vi "2048_summon_ani.vi"(6 "speed":u32, 8 "Array in":refnum<vi>, 9 "c":u64, 10 "r":u64, 11 "element":i32) -> ()   [LabVIEW 2021]
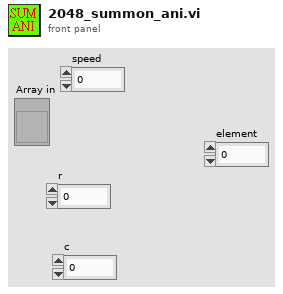
[diagram p1: front panel]
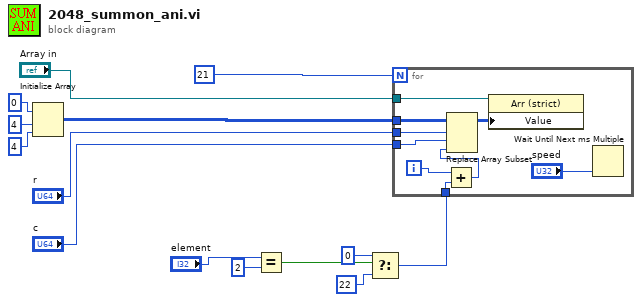
[diagram p0: block diagram]
diagram:
  n1 = Initialize Array(0 ("element"), 4 ("dimension size"), 4 ("dimension size")) -> (w14:i32[][])
  n2 = Equal?(x="element", y=2) -> (x = y?=w4:bool)
  n3 = Select(t=0, s=w4, f=22 ("t")) -> (s? t:f=w1:i32)
  n4 = for {
    N: 21 -> [_]
    tunnel: w14 -> [w23]
    tunnel: "c" -> [w21]
    tunnel: "r" -> [w20]
    tunnel: "Array in" -> [w19]
    tunnel: w1 -> [w17]
    i -> [w18]
    n5 = Add(x=w18, y=w17) -> (x+y=w16:i32)
    n6 = Replace Array Subset(array=w23, new element=w16, index (row)=w20, index (col)=w21) -> (w22:i32[][])
    n7 = property on="Property Node" class="Arr (strict)"(reference=w19, "Value"=w22) -> ()  [unwired: 1 in, 2 out]
    n8 = Wait Until Next ms Multiple(millisecond multiple="speed") -> ()  [unwired: 1 out]
  }
